vi "LNI Stufe testen.vi"(7 "Komponentenauswahl":T5 {"Konzentration" format="%#.6f"}, 8 "error in (no error)":errorcluster caption="Fehler (Eingang, kein Fehler)", 9 "Index Cluster":T4 {"Verdünnungsgas" items=["N2", "O2"]; "Anzahl Stufen" format="%#_5g"}, 11 "GD DIL Input":u16) -> (0 "error out":errorcluster caption="Fehler (Ausgang)", 2 "GD DF":T1, 3 "GD LNI old":T1)   [LabVIEW 2020, in "Linearisierung v2.lvlib" / "Gasteiler.lvlib"]
uses:
  Gasteiler.lvlib
  KomponentenArray.ctl
  Visualisierungs Elemente/Auswahlfeld.ctl
  Visualisierungs Elemente/Zahlen-Eingabefeld.ctl
  Visualisierungs Elemente/Checkbox(boolsch).ctl
  Aktionen FGV Gasteiler Daten.ctl
  SpanEinstellungen/Aktion FGV GD Errors sammeln.ctl
  SpanEinstellungen/GD Info Cluster.ctl
  LIN ErrorCluster.ctl
  Aktion FGV Gasteilerliste laden.ctl
  AK-Komm Gasteiler/Aktionen AK Komm.ctl
  AK-Komm Gasteiler/AK Komm Gasteiler.lvlib
  Aktion Lin Daten aufarbeiten.ctl
  Linearisierung v2.lvlib
  SpanEinstellungen/SpanEinstellungen.lvlib
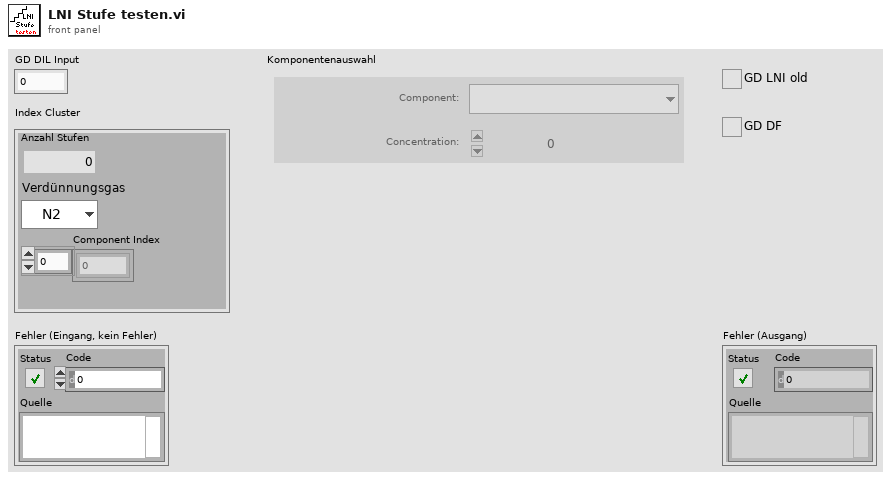
[diagram p1: front panel]
types:
  T1 = typedef "Checkbox(boolsch).ctl" = bool
  T2 = typedef "Zahlen-Eingabefeld.ctl" = sgl
  T3 = typedef "Linearisierung v2.lvlib/Gasteiler.lvlib/Prüfgas in.ctl" = u16
  T4 = cluster{"Anzahl Stufen":T2, "Verdünnungsgas":T3, "Component Index":i32[]}
  T5 = typedef "Linearisierung v2.lvlib/KomponentenArray.ctl" = cluster{"Komponente:":T6, "Konzentration":dbl}[]
  T6 = typedef "Auswahlfeld.ctl" = u16
  T7 = typedef "Linearisierung v2.lvlib/SpanEinstellungen.lvlib/GD Info Cluster.ctl" = cluster{"Wobei":string, "Status":string, "Errors":T8, "Empfangsdaten":string[], "Zeitstempel":string}
  T8 = typedef "Linearisierung v2.lvlib/LIN ErrorCluster.ctl" = cluster{"Störung Kommunikation":bool, "Pressure carrier gas":bool, "Pressure diluted gas":bool, "Outlet Pressure":bool, "SNOX before SAIR":bool, "Störung Gasteiler":bool}
  T9 = typedef "Linearisierung v2.lvlib/SpanEinstellungen.lvlib/Aktion FGV GD Errors sammeln.ctl" = enum16{"lesen", "init", "GD Infos sammeln", "Kalibrierinfos sammeln", "Test Data", "GD Infos selektiv sammeln"}
  T10 = typedef "Linearisierung v2.lvlib/Gasteiler.lvlib/Aktionen FGV Gasteiler Daten.ctl" = enum16{"lesen", "Gasteiler Daten", "Seriellen Param.", "MB-Endwert", "laden", "speichern", "Anforderung", "TCP", "Aufzeichnung Start"}
  T11 = typedef "Linearisierung v2.lvlib/Aktion Lin Daten aufarbeiten.ctl" = enum16{"lesen", "Protkolldaten", "speichern", "laden", "EPA auswerten", "Tabelle schreiben", "Lin auswerten", "Tab init", "Stufentabelle", "EPA aktiviert", "Nachbehandlung laden", "Tabelle löschen", "Istwerte löschen", "Zeile löschen", "Zeile einfügen", "LIN aktiviert", "LIN/EPA aktiv laden", "EGAK Tab", "LIN übernehmen", "Tab init ohne Stufen"}
  T12 = typedef "Linearisierung v2.lvlib/Lin-Polynom Daten.ctl" = cluster{"Messgerät":string, "Kalibrator (Gasteiler)":string, "Bearbeiter/in":string, "Komponente":string, "Zeitstempel":timestamp, "F_max gefordert (%)":sgl, "F_max in %":sgl, "F_max in ppm":sgl, "Vorschlag Ordnung":i32, "Polynom OK":bool, "Polynomkoeff.":dbl[], "Prüfgas Konzentration":dbl, "Pfad EPA":string, "Pfad_LIN":string, "Gasnummer:":u8, "Komponentenauswahl":T5, "Verdünnungsgas":T3, "Zeitdauer Stufe":T2, "Anzahl Stufen":T2, "F_max in % EPA":sgl, "F_max in ppm EPA":sgl, "F_max in % LIN":sgl, "F_max in ppm LIN":sgl, "Punkte umkehren":bool, "EPA Optionsfeld":T13, "Autolin Hovacal":T14, "Spanfactors":sgl[], "Kalibrierauswahl":T15, "Conditions:":T16, "Gasflaschen Nr.:":string, "Bottle Accuracy":dbl, "Konfig Gasflasche":T17, "Gasflasche":T18, "HovaCAL Flow AutoLin":T19, "MFC Output":T20, "Gas Ablaufdatum":timestamp, "Lin Modus":T21, "zusätzliche Zeitdauer Erster Punkt":sgl, "Offsets":sgl[]}
  T13 = typedef "Linearisierung v2.lvlib/EPA Optionsfeld.ctl" = enum32{"Istwert", "Rohwert", "Linearisierter Wert"}
  T14 = typedef "Linearisierung v2.lvlib/Gasteiler.lvlib/HovaCal.lvlib/AutoLin Hovacal.ctl" = enum32{"Keine Auswahl", "Optionsauswahl 1", "Optionsauswahl 2"}
  T15 = typedef "Linearisierung v2.lvlib/Kalibrieroption.ctl" = u16
  T16 = typedef "Linearisierung v2.lvlib/Linearity verification 1065-307.lvlib/Condition.ctl" = u16
  T17 = typedef "System Einstellungen V2.lvlib/Konfig Gasflasche.ctl" = bool
  T18 = typedef "System Einstellungen V2.lvlib/Gasflasche Auswahl.ctl" = u16
  T19 = typedef "Linearisierung v2.lvlib/Gasteiler.lvlib/HovaCAL_Interface.lvlib/Controls.lvlib/Flow Einstellung.ctl" = cluster{"HovaCAL Flow Input Cluster":dbl}
  T20 = typedef "Linearisierung v2.lvlib/Gasteiler.lvlib/HovaCAL_Interface.lvlib/Controls.lvlib/Pump state.ctl" = cluster{"Run":bool}
  T21 = typedef "Linearisierung v2.lvlib/Lin Modus.ctl" = u16
  T22 = typedef "Linearisierung v2.lvlib/Gasteiler.lvlib/Aktion FGV Gasteilerliste laden.ctl" = enum16{"lesen", "laden", "speichern", "Liste erstellen", "Formel ändern", "Gas vereinzeln"}
  T23 = typedef "Linearisierung v2.lvlib/Gasteiler.lvlib/Gasteiler Daten.ctl" = cluster{"Gasteiler":T24, "Gasteiler Stufen":T25, "Gasteiler Type":T26, "Konfig Gasteiler":T27, "Gasteiler Span Eingänge":u16}
  T24 = typedef "String - Eingabefeld.ctl" = string
  T25 = typedef "Linearisierung v2.lvlib/Gasteiler.lvlib/Gasteiler Stufen.ctl" = u16
  T26 = typedef "Linearisierung v2.lvlib/GasteilerType.ctl" = u16
  T27 = typedef "System Einstellungen V2.lvlib/Gasteiler Auswahl.ctl" = u16
  T28 = typedef "Linearisierung v2.lvlib/Gasteiler.lvlib/AK Komm Gasteiler.lvlib/Aktionen AK Komm.ctl" = enum16{"lesen", "initialisieren", "beenden", "Status", "SMAN", "SREM", "STBY", "ASTF", "ASTZ", "SLST", "AGAT", "EGAK", "AGAK", "AKAK", "ADRU", "SKOP", "SVSA", "SVSZ", "SONO", "SAIR", "SNOX", "ANOX", "SSPL", "SRUC", "SLIN", "ALST", "ETYP", "SVIO", "LCYL", "CCYL", "DCYL", "SCYL", "GCYL", "DRGV", "DRDC"}
  T29 = typedef "System Einstellungen V2.lvlib/Traegergas.ctl" = string
  T30 = typedef "Linearisierung v2.lvlib/Gasteiler.lvlib/Gasteiler Fehler.ctl" = cluster{"Pressure carrier gas":bool, "Pressure diluted gas":bool, "Outlet Pressure":bool, "SNOX before SAIR":bool}
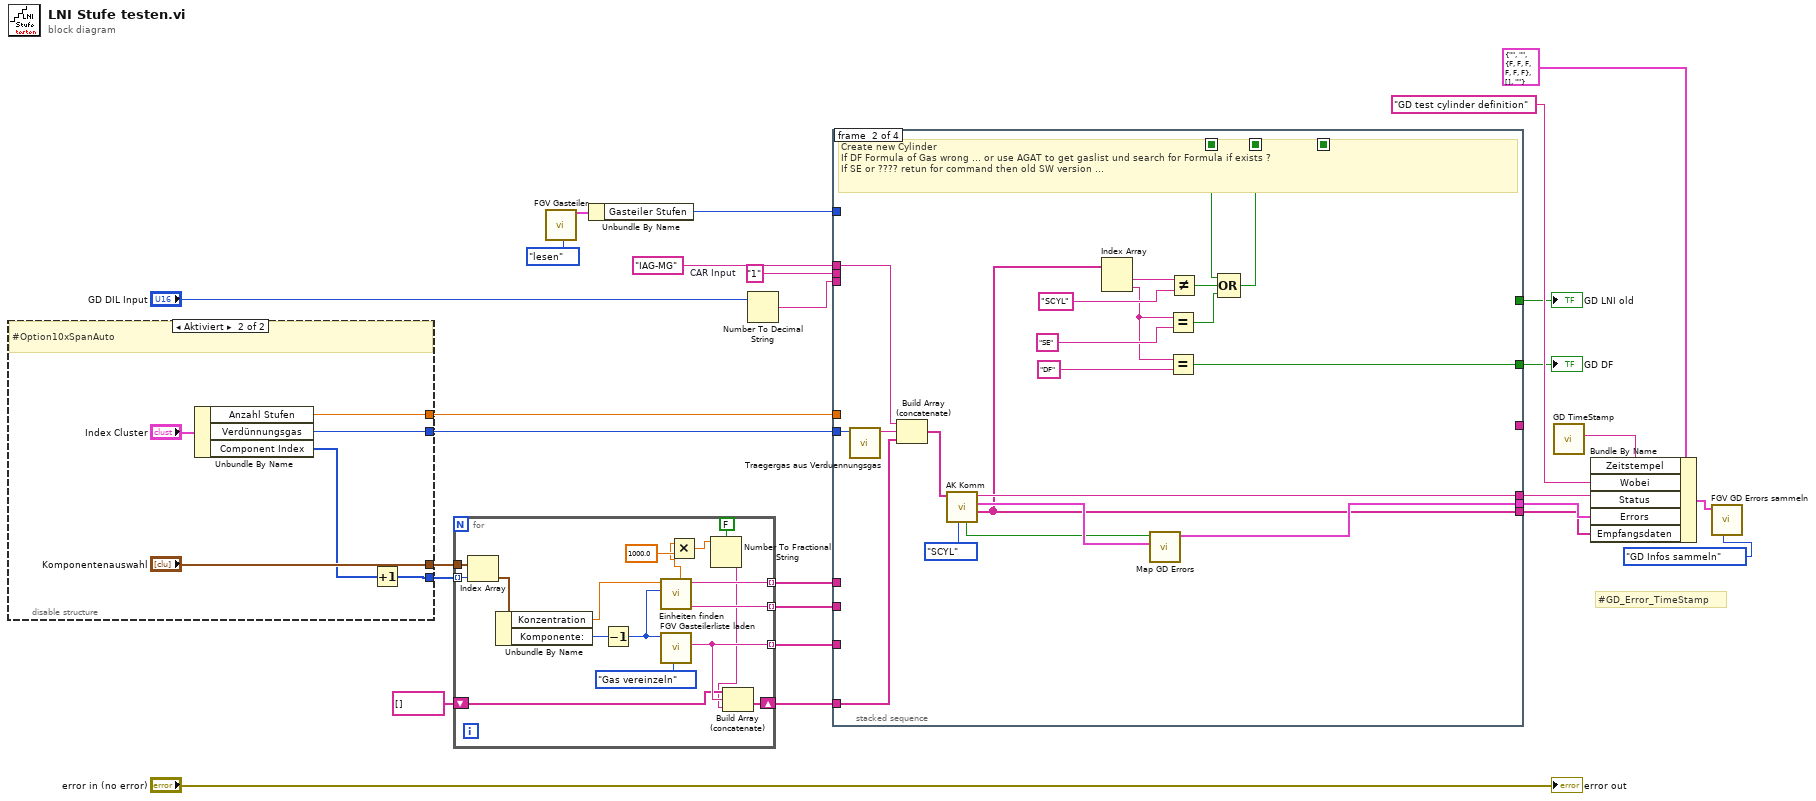
[diagram p0: block diagram]
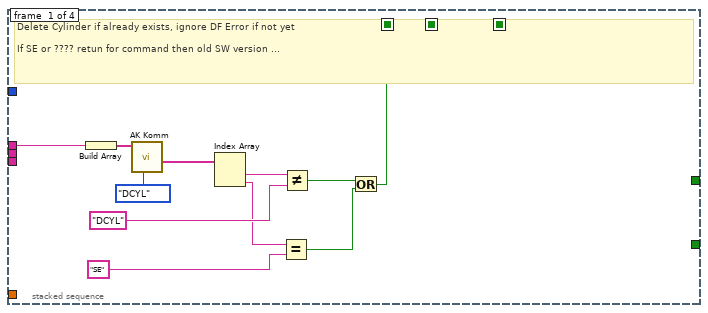
[diagram p2: hidden frame]
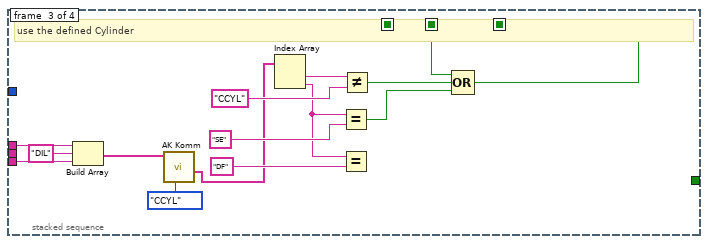
[diagram p3: hidden frame]
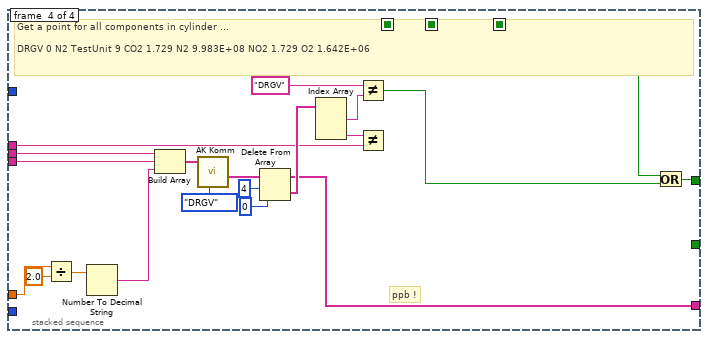
[diagram p4: hidden frame]
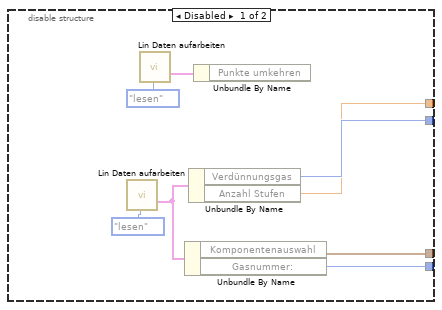
[diagram p5: hidden frame]
diagram:
  w4 = "1"  # CAR Input
  # "#GD_Error_TimeStamp"
  n1 = disable-structure shown="Aktiviert" {
    disable-tunnel: [w35 "Komponentenauswahl"] -> w24
    disable-tunnel: [w34 w39] -> w26
    disable-tunnel: [w32 w40] -> w25
    disable-tunnel: [w28 w37] -> w23
    frame Disabled {
      n2 = call "Lin Daten aufarbeiten.vi"("Aktionen"=Aktion_Lin_Daten_aufarbeiten."lesen") -> ("Lin-Polynom"=w33:T12)  [unwired: 16 in, 10 out]
      n3 = call "Lin Daten aufarbeiten.vi"("Aktionen"=Aktion_Lin_Daten_aufarbeiten."lesen") -> ("Lin-Polynom"=w30:T12)  [unwired: 16 in, 10 out]
      n4 = Unbundle By Name(w33) -> ("Komponentenauswahl"=w35:T5, "Gasnummer:"=w28:u8)
      n5 = Unbundle By Name(w33) -> ("Verdünnungsgas"=w34:T3, "Anzahl Stufen"=w32:T2)
      n6 = Unbundle By Name(w30) -> ("Punkte umkehren"=w29:bool)
    }
    frame Enabled {
      # "#Option10xSpanAuto"
      n7 = Unbundle By Name("Index Cluster") -> ("Anzahl Stufen"=w40:T2, "Verdünnungsgas"=w39:T3, "Component Index"=w38:i32[])
      n8 = Increment(x=w38) -> (x+1=w37:i32[])
    }
  }
  n9 = for {
    tunnel: w24 -> [w59]
    tunnel: w23 -> [w58] mode=indexing
    tunnel: [w51] -> w22 mode=indexing
    tunnel: [w52] -> w21 mode=indexing
    shift-right: [w50] -> w9
    shift-left: string[] [] -> [w49]
    tunnel: [w48] -> w5 mode=indexing
    n10 = Index Array(array=w59, index=w58) -> (element=w56:cluster{"Komponente:":T6, "Konzentration":dbl})
    n11 = Unbundle By Name(w56) -> ("Konzentration"=w53:dbl, "Komponente:"=w55:T6)
    n12 = Decrement(x=w55) -> (x-1=w54:T6)
    n13 = call "Einheiten finden.vi"("Komponente"=w54, "Wert"=w53) -> ("Einheit in String"=w48:string, "String"=w51:string, "Wert ppm"=w44:dbl)  [unwired: 5 in, 2 out]
    n14 = call "FGV Gasteilerliste laden.vi"("Aktion"=Aktion_FGV_Gasteilerliste_laden."Gas vereinzeln", "Gasindex"=w54) -> ("Formel"=w52:string)  [unwired: 7 in, 2 out]
    n15 = Multiply(x=w44, y=1000.0) -> (x*y=w46:dbl)
    n16 = Number To Fractional String(use system decimal point (T)=FALSE ("Systemdezimalzeichen verwenden (T)"), number=w46) -> (F-format string=w43:string)  [unwired: 2 in]
    n17 = Build Array (concatenate)(w49, w52, w43) -> (w50:string[])
  }
  n18 = call "FGV Gasteiler.vi"("Aktionen"=Aktionen_FGV_Gasteiler_Daten."lesen") -> ("Gasteiler Daten"=w20:T23)  [unwired: 11 in, 7 out]
  n19 = Unbundle By Name(w20) -> ("Gasteiler Stufen"=w18:T25)
  n20 = Number To Decimal String(number="GD DIL Input") -> (decimal integer string=w2:string)  [unwired: 1 in]
  n21 = stacked-sequence {
    seq-local: [w60 _ _ _] -> [_ w72 _ _]
    seq-local: [_ w71 _ _] -> [_ _ w94 _]
    seq-local: [_ _ w93 _] -> [_ _ _ w113]
    tunnel: w22 -> [_ _ _ _]
    tunnel: w21 -> [_ _ _ _]
    tunnel: w18 -> [_ _ _ _]
    tunnel: w26 -> [_ w90 _ _]
    tunnel: w25 -> [_ _ _ w125]
    tunnel: [_ w87 _ _] -> w14
    tunnel: [_ w79 _ _] -> w12
    tunnel: [_ w85 _ _] -> w13
    tunnel: "IAG-MG" -> [w69 w83 w104 w111]
    tunnel: w9 -> [_ w82 _ _]
    tunnel: [_ _ _ w115] -> w7
    tunnel: [_ w73 _ _] -> w6
    tunnel: w5 -> [_ _ _ _]
    tunnel: [_ _ _ w109] -> _
    tunnel: w4 -> [_ _ _ w108]
    tunnel: w2 -> [_ _ w92 w107]
    frame #0 {
      # "Delete Cylinder if already exists, ignore DF Error if not yet\n\nIf SE or ???? retun for command then old SW version ..."
      n22 = Build Array(w69) -> (w68:string[])
      n23 = call "AK Komm.vi"("Aktionen"=Aktionen_AK_Komm."DCYL", "Daten"=w68) -> ("Empfangsdaten"=w67:string[])  [unwired: 3 in, 6 out]
      n24 = Index Array(array=w67) -> (element #1=w66:string, element #2=w63:string)  [unwired: 2 in]
      n25 = Equal?(x=w63, y="SE") -> (x = y?=w61:bool)
      n26 = Not Equal?(x=w66, y="DCYL") -> (x != y?=w64:bool)
      n27 = Or(x=w64, y=w61) -> (x .or. y?=w60:bool)
    }
    frame #1 {
      # "Create new Cylinder \nIf DF Formula of Gas wrong ... or use AGAT to get gaslist und search for Formula if exists ?\nIf SE or ???? retun for command then old SW version ..."
      n28 = call "Traegergas aus Verduennungsgas.vi"("Verdünnungsgas"=w90) -> ("Trägergas"=w89:T29)  [unwired: 10 in]
      n29 = Build Array (concatenate)(w83, w89, w82) -> (w88:T29[])
      n30 = call "AK Komm.vi"("Aktionen"=Aktionen_AK_Komm."SCYL", "Daten"=w88) -> ("Empfangsdaten"=w79:string[], "Error"=w86:T30, "Status"=w87:string, "Störung Kommunikation"=w84:bool)  [unwired: 3 in, 3 out]
      n31 = Index Array(array=w79) -> (element #1=w81:string, element #2=w77:string)  [unwired: 2 in]
      n32 = call "Map GD Errors.vi"("Error"=w86, "Störung Kommunikation"=w84) -> ("LIN Errors-Cluster (Ausgang)"=w85:T8)  [unwired: 8 in, 1 out]
      n33 = Equal?(x=w77, y="SE") -> (x = y?=w74:bool)
      n34 = Equal?(x=w77, y="DF") -> (x = y?=w73:bool)
      n35 = Not Equal?(x=w81, y="SCYL") -> (x != y?=w75:bool)
      n36 = Compound Arithmetic op=OR ("Mehrfacharithmetik")(w72, w75, w74) -> (w71:bool)
    }
    frame #2 {
      # "use the defined Cylinder"
      n37 = Build Array(w104, "DIL", w92) -> (w105:string[])
      n38 = call "AK Komm.vi"("Aktionen"=Aktionen_AK_Komm."CCYL", "Daten"=w105) -> ("Empfangsdaten"=w95:string[])  [unwired: 3 in, 6 out]
      n39 = Index Array(array=w95) -> (element #1=w102:string, element #2=w99:string)  [unwired: 2 in]
      n40 = Equal?(x=w99, y="SE") -> (x = y?=w96:bool)
      n41 = Equal?(x=w99, y="DF") -> ()  [unwired: 1 out]
      n42 = Not Equal?(x=w102, y="CCYL") -> (x != y?=w97:bool)
      n43 = Compound Arithmetic op=OR ("Mehrfacharithmetik")(w94, w97, w96) -> (w93:bool)
    }
    frame #3 {
      # "ppb !"
      # "Get a point for all components in cylinder ...\n\nDRGV 0 N2 TestUnit 9 CO2 1.729 N2 9.983E+08 NO2 1.729 O2 1.642E+06"
      n44 = Divide(x=w125, y=T2 2.0) -> (x/y=w123:T2)
      n45 = Number To Decimal String(number=w123) -> (decimal integer string=w122:string)  [unwired: 1 in]
      n46 = Build Array(w108, w107, w122) -> (w121:string[])
      n47 = call "AK Komm.vi"("Aktionen"=Aktionen_AK_Komm."DRGV", "Daten"=w121) -> ("Empfangsdaten"=w110:string[])  [unwired: 3 in, 6 out]
      n48 = Delete From Array(array=w110, length=4 ("Länge"), index=0 ("Index")) -> (deleted portion=w118:string[], array with subset deleted=w109:string[])
      n49 = Index Array(array=w118) -> (element #1=w116:string, element #3=w112:string)  [unwired: 3 in, 1 out]
      n50 = Not Equal?(x="DRGV", y=w116) -> (x != y?=w114:bool)
      n51 = Not Equal?(x=w112, y=w111) -> ()  [unwired: 1 out]
      n52 = Or(x=w113, y=w114) -> (x .or. y?=w115:bool)
    }
  }
  "GD LNI old" <- w7
  "GD DF" <- w6
  n53 = call "GD TimeStamp.vi"() -> ("date/time string"=w1:string)  [unwired: 10 in, 1 out]
  n54 = Bundle By Name(cluster=T7 {"Wobei"="", "Status"="", "Errors"={"Störung Kommunikation"=FALSE, "Pressure carrier gas"=FALSE, "Pressure diluted gas"=FALSE, "Outlet Pressure"=FALSE, "SNOX before SAIR"=FALSE, "Störung Gasteiler"=FALSE}, "Empfangsdaten"=[], "Zeitstempel"=""} ("GD Info-Cluster"), "Zeitstempel"=w1, "Wobei"="GD test cylinder definition" ("Status"), "Status"=w14, "Errors"=w13, "Empfangsdaten"=w12) -> (w11:T7)
  n55 = call "FGV GD Errors sammeln.vi"("Aktion"=Aktion_FGV_GD_Errors_sammeln."GD Infos sammeln", "GD Info-Cluster in"=w11) -> ()  [unwired: 7 in, 3 out]
  "error out" <- "error in (no error)"
